vi "Host__MainNew.vi"() -> ()   [LabVIEW 2018]
uses:
  HealthCheckClass/HealthCheck.lvclass
panel:
  in  "Tab Control":enum32{"Page 1", "Page 2"}(tab)
  in  "Edit Table":bool
  out "HealthCheckTable":string[][](table)
  in  "stop":bool
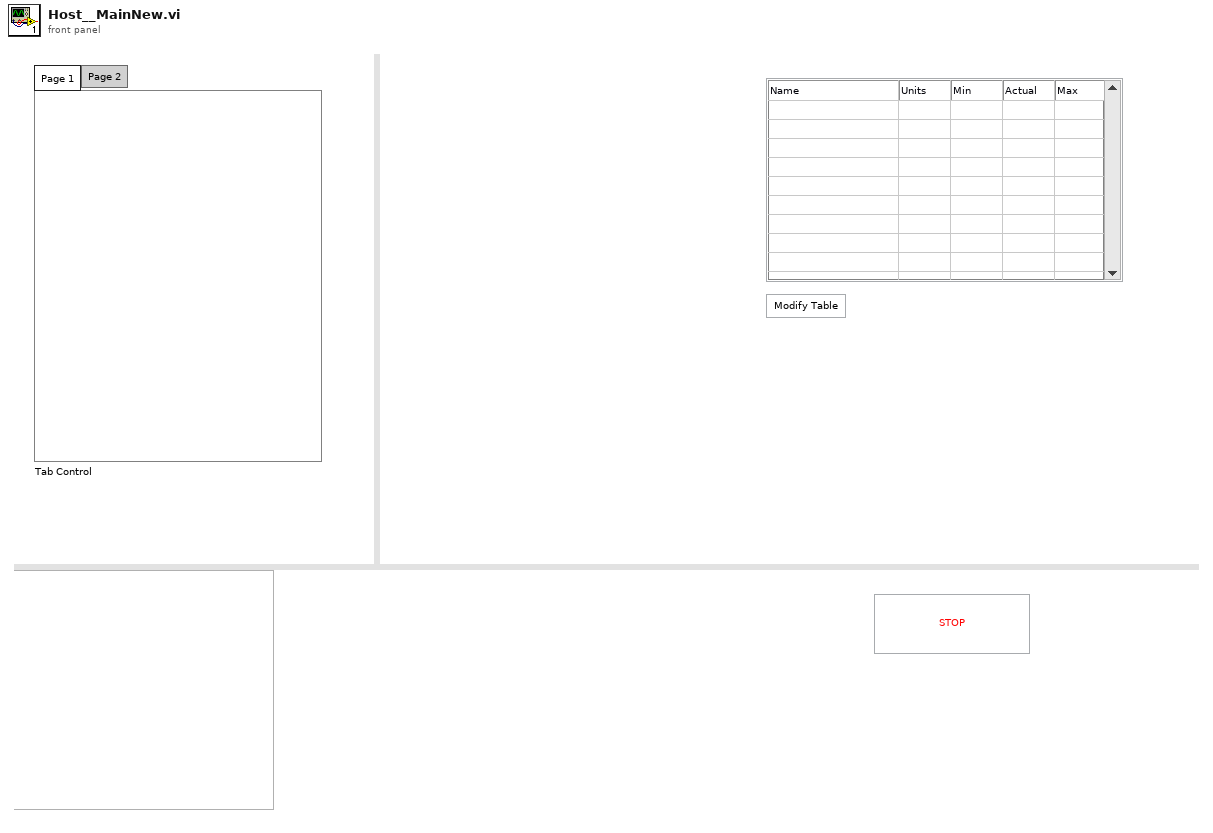
[diagram p1: front panel]
types:
  T1 = typedef "HealthCheck.lvclass/HCState_TypeDef.ctl" = enum16{"Initialization", "Running", "Modify Table"}
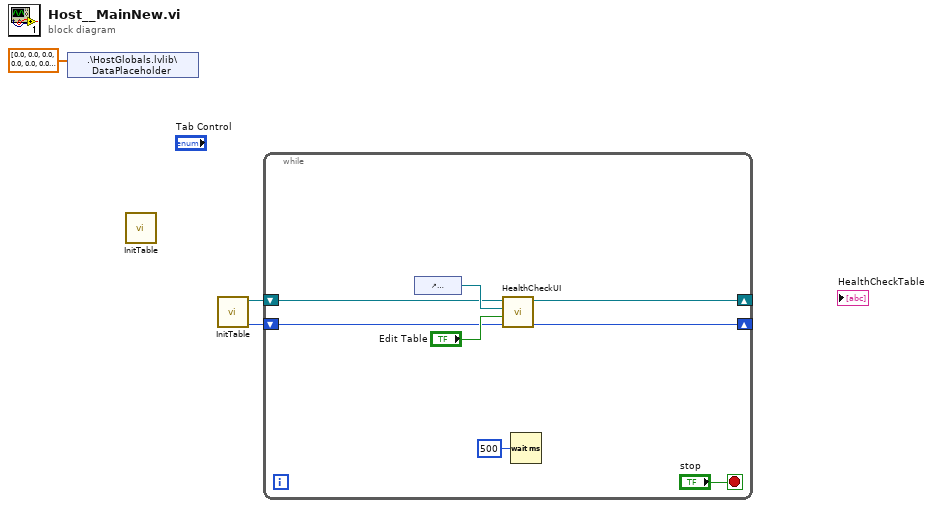
[diagram p0: block diagram]
diagram:
  n1 = shared-variable ".\\HostGlobals.lvlib\\DataPlaceholder"(dbl[] [0.0, 0.0, 0.0, 0.0, 0.0, 0.0, 0.0, 0.0, 0.0, 0.0] ("DataPlaceholder")) -> ()  [unwired: 1 in, 1 out]
  n2 = call "InitTable.vi"() -> ()  [unwired: 10 in, 2 out]
  n3 = call "InitTable.vi"() -> ("Enum out"=w1:T1, "HealthCheck out"=w2:refnum<class "HealthCheck.lvclass">)  [unwired: 10 in]
  n4 = while {
    shift-right: [w7] -> _
    shift-left: w2 -> [w6]
    shift-right: [w5] -> _
    shift-left: w1 -> [w4]
    stop <- "stop" stop-if-true
    n5 = control-ref of="HealthCheckTable"() -> (w8:refnum<vi>)
    n6 = call "HealthCheckUI.vi"("Enum in"=w4, "Edit Table"="Edit Table", "Table in"=w8, "HealthCheck.lvclass"=w6) -> ("Enum out"=w5:T1, "HealthCheck out"=w7:refnum<class "HealthCheck.lvclass">)  [unwired: 6 in]
    n7 = Wait (ms)(milliseconds to wait=u32 500) -> ()  [unwired: 1 out]
  }
